vi "sub 1.vi"(8 "error in (no error)":errorcluster, 11 "Numeric":i32) -> (0 "error out":errorcluster, 3 "Sine":dbl)   [LabVIEW 2015]
uses:
  <vilib>/ptbypt/NI_PtbyPt.lvlib
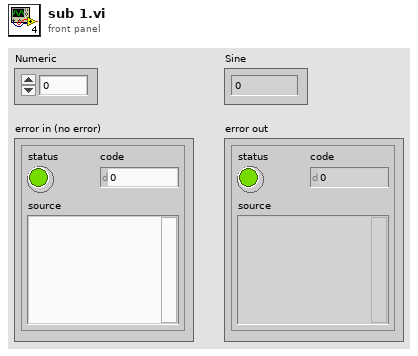
[diagram p1: front panel]
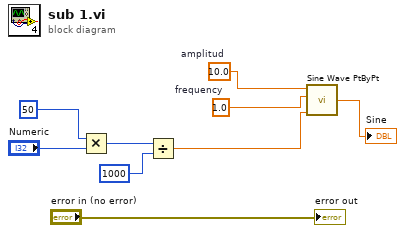
[diagram p0: block diagram]
diagram:
  w2 = 1.0  # frequency
  w3 = 10.0  # amplitud
  n1 = Multiply(x=50, y="Numeric") -> (x*y=w6:i32)
  n2 = Divide(x=w6, y=1000) -> (x/y=w1:dbl)
  n3 = call <vilib>:"Sine Wave PtByPt.vi"("time"=w1, "frequency"=w2, "amplitude"=w3) -> ("sine wave"=→"Sine":dbl)  [unwired: 1 in]
  "error out" <- "error in (no error)"
